vi "ROI 2 INI Section.vi"(7 "section":string="ROI", 8 "error in (no error)":errorcluster, 10 "ROI Descriptor":T2 {"Contours"."Type" items=["No Selection", "Point", "Line", "Rectangle", "Oval", "Polygon", "Freehand Region", "Annulus", "Unused2", "Unused3", "Broken Line", "Freehand Line", "Rotated Rectangle"]}, 11 "refnum in":T1) -> (0 "error out":errorcluster, 3 "refnum out":T1)   [LabVIEW 2020, in "POLARIS Vision utility.lvlib"]
uses:
  POLARIS Vision utility.lvlib
  <vilib>/Utility/config.llb/Config Data RefNum.ctl
  <vilib>/Utility/config.llb/Write Key (I32).vi
  <vilib>/Utility/config.llb/Write Key (U32).vi
  <vilib>/Utility/config.llb/NI_LVConfig.lvlib
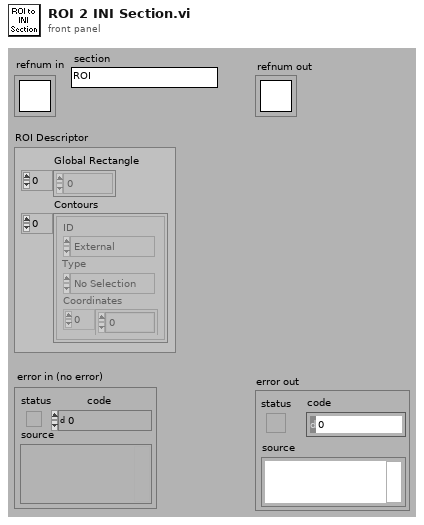
[diagram p1: front panel]
types:
  T1 = typedef "NI_LVConfig.lvlib/Config Data RefNum.ctl" = refnum<k1>
  T2 = typedef "ROI Descriptor" = cluster{"Global Rectangle":i32[], "Contours":cluster{"ID":enum32{"External", "Internal"}, "Type":u32, "Coordinates":i32[]}[]}
  T3 = cluster{"ID":enum32{"External", "Internal"}, "Type":u32, "Coordinates":i32[]}[]
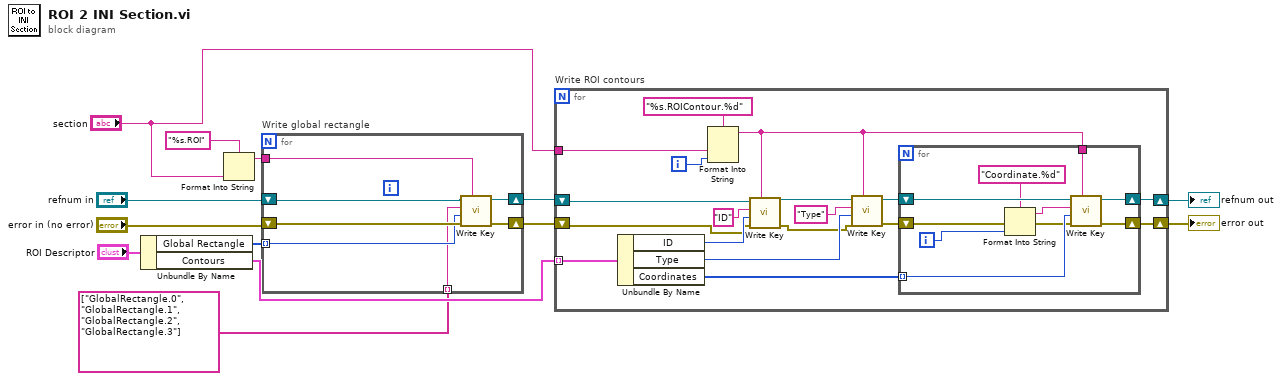
[diagram p0: block diagram]
diagram:
  n1 = Unbundle By Name("ROI Descriptor") -> ("Global Rectangle"=w8:i32[], "Contours"=w12:T3)
  n2 = Format Into String(format string="%s.ROI", "section") -> (resulting string=w1:string)  [unwired: 2 in, 1 out]
  n3 = for "Write global rectangle" {
    shift-right: [w19] -> w7
    shift-left: "error in (no error)" -> [w20]
    shift-right: [w17] -> w9
    shift-left: "refnum in" -> [w18]
    tunnel: w8 -> [w16] mode=indexing
    tunnel: string[] ["GlobalRectangle.0", "GlobalRectangle.1", "GlobalRectangle.2", "GlobalRectangle.3"] -> [w15] mode=indexing
    tunnel: w1 -> [w14]
    n4 = call-poly <vilib>:"Write Key.vi"("section"=w14, "error in (no error)"=w20, "value"=w16, "key"=w15, "refnum"=w18) -> ("error out"=w19:errorcluster, "refnum out"=w17:T1)  [unwired: 4 in, 1 out]
  }
  n5 = for "Write ROI contours" {
    tunnel: w12 -> [w38] mode=indexing
    shift-right: [w26] -> w10
    shift-left: w9 -> [w36]
    shift-right: [w25] -> w11
    shift-left: w7 -> [w27]
    tunnel: "section" -> [w22]
    i -> [w21]
    n6 = Unbundle By Name(w38) -> ("ID"=w35:enum32{"External", "Internal"}, "Type"=w31:u32, "Coordinates"=w37:i32[])
    n7 = Format Into String(format string="%s.ROIContour.%d" ("section"), w22, w21) -> (resulting string=w24:string)  [unwired: 2 in, 1 out]
    n8 = call-poly <vilib>:"Write Key.vi"("section"=w24, "error in (no error)"=w27, "value"=w35, "key"="ID", "refnum"=w36) -> ("error out"=w30:errorcluster, "refnum out"=w33:T1)  [unwired: 4 in, 1 out]
    n9 = call-poly <vilib>:"Write Key.vi"("section"=w24, "error in (no error)"=w30, "value"=w31, "key"="Type", "refnum"=w33) -> ("error out"=w28:errorcluster, "refnum out"=w29:T1)  [unwired: 4 in, 1 out]
    n10 = for {
      tunnel: w37 -> [w46] mode=indexing
      tunnel: w24 -> [w47]
      shift-right: [w45] -> w25
      shift-left: w28 -> [w40]
      shift-right: [w44] -> w26
      shift-left: w29 -> [w48]
      i -> [w43]
      n11 = Format Into String(format string="Coordinate.%d" ("string"), error in=w40, w43) -> (resulting string=w41:string, error out=w39:errorcluster)  [unwired: 1 in]
      n12 = call-poly <vilib>:"Write Key.vi"("section"=w47, "error in (no error)"=w39, "value"=w46, "key"=w41, "refnum"=w48) -> ("error out"=w45:errorcluster, "refnum out"=w44:T1)  [unwired: 4 in, 1 out]
    }
  }
  "error out" <- w11
  "refnum out" <- w10
